vi "CSM - Start Watchdog to Ensure All Modules Exit.vi"(6 "Wait(5000ms)":i32=5000, 8 "error in (no error)":errorcluster) -> (0 "error out":errorcluster)   [LabVIEW 2017, in "CSM Watchdog.lvlib"]
doc: "Starts the CSM Watchdog thread to monitor whether the main program has exited. It is typically executed immediately after the main program starts.\n\n<b>Application Scenario</b>: Used to ensure that all asynchronously started CSM modules can exit normally after the main program exits.\n\n\n> [!NOTE] <b>CSM WatchDog Implementation Principle</b>\n>\n> When a LabVIEW VI exits, it automatically releases all handle resources such as queues and events. Therefore, you can create a WatchDog thread that monitors a queue resource created by the main program VI. When this queue resource is released after the main VI exits, the WatchDog thread is triggered to send `Macro: Exit` to any CSM modules that have not yet exited, ensuring they exit normally.\n\n\n-- <b>Controls</b> --\n- <b>Wait(5000ms)</b>: The time the Watchdog thread waits for modules to process `Macro: Exit` and exit, in milliseconds (ms). The default value is 5000 ms."
uses:
  CSM Watchdog.lvlib
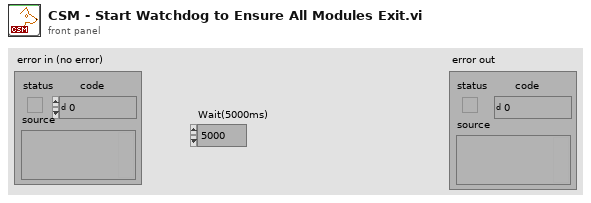
[diagram p1: front panel]
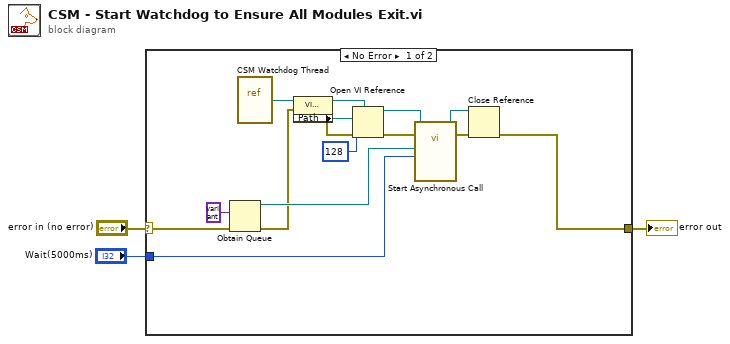
[diagram p0: block diagram]
diagram:
  n1 = case shown="No Error" "error in (no error)" {
    selector: "error in (no error)" -> [w6 w19]
    tunnel: [w9 w19] -> w2
    tunnel: "Wait(5000ms)" -> [w4 _]
    frame No Error {
      n2 = Obtain Queue(element data type=variant, error in (no error)=w6) -> (queue out=w7:refnum<queue>, error out=w5:errorcluster)  [unwired: 3 in, 1 out]
      n3 = vi-ref "CSM Watchdog Thread.vi"() -> (w12:refnum<vi>)
      n4 = property class="VI (strict)"(reference=w12, error in=w5) -> (reference out=w16:refnum<vi>, error out=w14:errorcluster, "Path"=w13:path)
      n5 = Open VI Reference(type specifier VI Refnum (for type only)=w16, vi path=w13, options=128, error in (no error)=w14) -> (vi reference=w11:refnum<vi>, error out=w17:errorcluster)  [unwired: 2 in]
      n6 = call-by-ref "Start Asynchronous Call"(reference=w11, error in=w17, "Wait(5000ms)"=w4, "Watchdog Queue"=w7) -> (reference out=w10:refnum<vi>, error out=w15:errorcluster)  [unwired: 10 in]
      n7 = Close Reference(reference=w10, error in (no error)=w15) -> (error out=w9:errorcluster)
    }
    frame Error {
    }
  }
  "error out" <- w2
